vi "setLoadImpedance.vi"(8 "error in (no error)":errorcluster, 10 "Load Impedance":T1 items=["50 Ohm"=50.0, "High Z"=10000000.0], 11 "FgenKeysight in":refnum<class "ArbKeysight.lvclass">) -> (0 "error out":errorcluster, 3 "FgenKeysight out":refnum<class "ArbKeysight.lvclass">)   [LabVIEW 2023, in "ArbKeysight.lvclass"]
doc: "<b>Author:</b> Wolfgang\n<b>Description:</b> Specify the output load impendance. 50 Ohms, HighZ => 10 M"
uses:
  ArbKeysight.lvclass
  Data/arbLoadImpedance.ctl
  ArbKeysight.lvclass/ArbKeysight.ctl
  Arb.lvclass
  Driver/Keysight-33500B.lvlib
  sweArb.lvlib
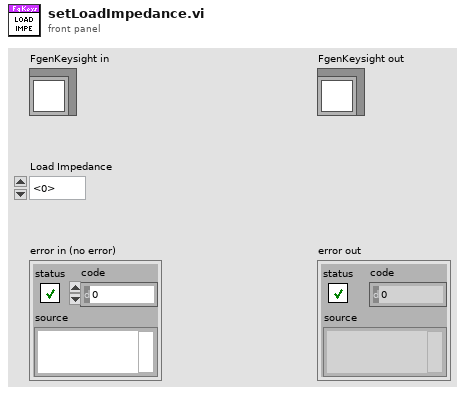
[diagram p1: front panel]
types:
  T1 = typedef "sweArb.lvlib/arbLoadImpedance.ctl" = dbl
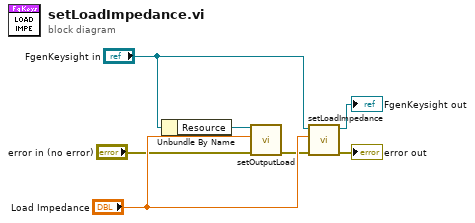
[diagram p0: block diagram]
diagram:
  n1 = Unbundle By Name("FgenKeysight in") -> ("Resource"=w4:refnum<visa-resource-name>)
  n2 = call "setOutputLoad.vi"("error in (no error)"="error in (no error)", "Phase"="Load Impedance", "VISA resource name"=w4) -> ("error out"=w1:errorcluster)  [unwired: 7 in, 1 out]
  n3 = call-parent "setLoadImpedance.vi"("error in (no error)"=w1, "Load Impedance"="Load Impedance", "Fgen in"="FgenKeysight in") -> ("error out"=→"error out":errorcluster, "Fgen out"=→"FgenKeysight out":refnum<class "ArbKeysight.lvclass">)  [unwired: 7 in]
